vi "GT Ln XY Override2.vi"(0 "cardNum":i16, 1 "synVel":dbl, 2 "velEnd":dbl, 5 "crd":i16, 7 "x":i32, 9 "y":i32, 11 "error in (no error)":errorcluster caption="错误输入（无错误）", 12 "synAcc":dbl, 13 "fifo":i16) -> (4 "function return":i16, 15 "error out":errorcluster caption="错误输出")   [LabVIEW 2020, in "gts.lvlib"]
doc: "GT_API GT_LnXYOverride2(short cardNum,short crd,long x,long y,double synVel,double synAcc,double velEnd=0,short fifo=0);"
uses:
  gts.lvlib
  dll/32bit/multi_card/gts.dll
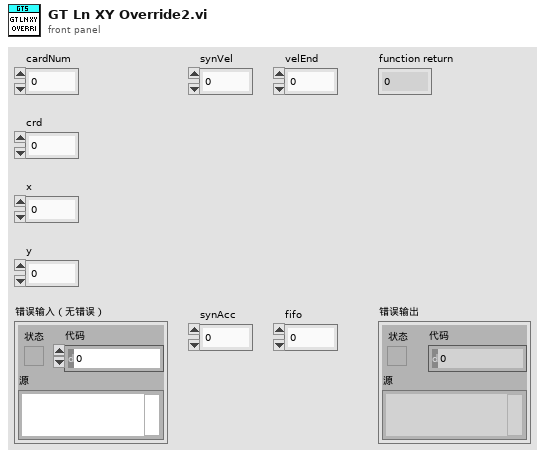
[diagram p1: front panel]
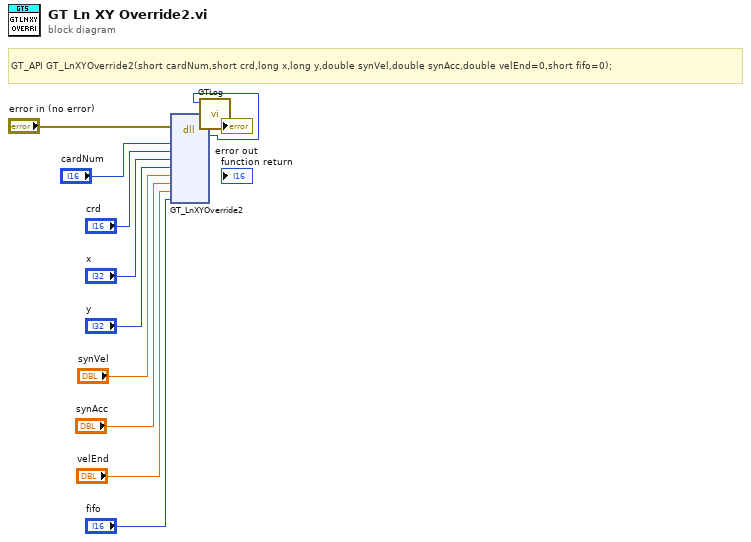
[diagram p0: block diagram]
diagram:
  # "GT_API GT_LnXYOverride2(short cardNum,short crd,long x,long y,double synVel,double synAcc,double velEnd=0,short fifo=0);"
  n1 = dll-call lib="C:/1228/dll/32bit/multi_card/gts.dll" fn="GT_LnXYOverride2"(error in="error in (no error)", "cardNum"="cardNum", "crd"="crd", "x"="x", "y"="y", "synVel"="synVel", "synAcc"="synAcc", "velEnd"="velEnd", "fifo"="fifo") -> (error out=w3:errorcluster, w1:i16)  [unwired: 10 in, 1 out]
  n2 = call "GTLog.vi"("error in (no error)"=w3, "Numeric"=w1) -> ("error out"=→"error out":errorcluster)  [unwired: 9 in]
